vi "Enqueue Message (Single).vi"(6 "Priority Message? (F)":bool, 8 "error in (no error)":errorcluster[](array[cluster]), 9 "Message Data":variant, 10 "Message":string, 11 "Message Queue":refnum<queue>) -> (0 "error out":errorcluster[](array[cluster]), 3 "dup Message Queue":refnum<queue>)   [LabVIEW 2018, in "Message Queue.lvlib"]
doc: "For a regular message, enqueue the message. For a priority message, enqueue it at the front of the queue."
uses:
  Message Queue.lvlib
  Message Cluster.ctl
  <userlib>/NIST/NISTErrorLib/NISTErrorLib.lvlib
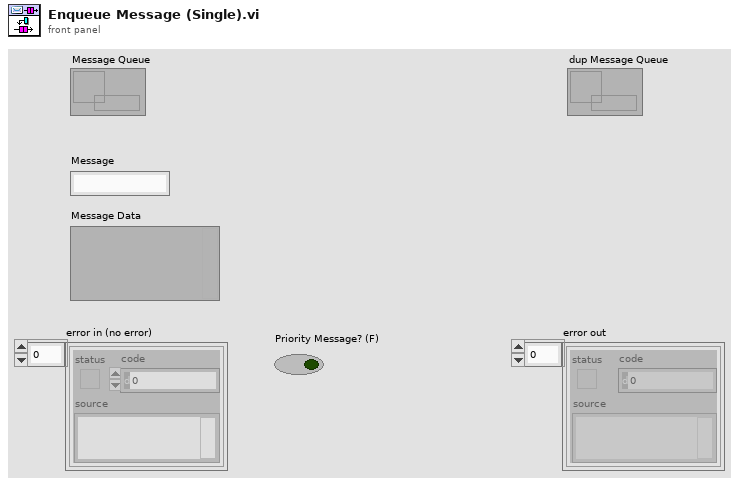
[diagram p1: front panel]
types:
  T1 = typedef "Message Queue.lvlib/Message Cluster.ctl" = cluster{"Message":string, "Message Data":variant}
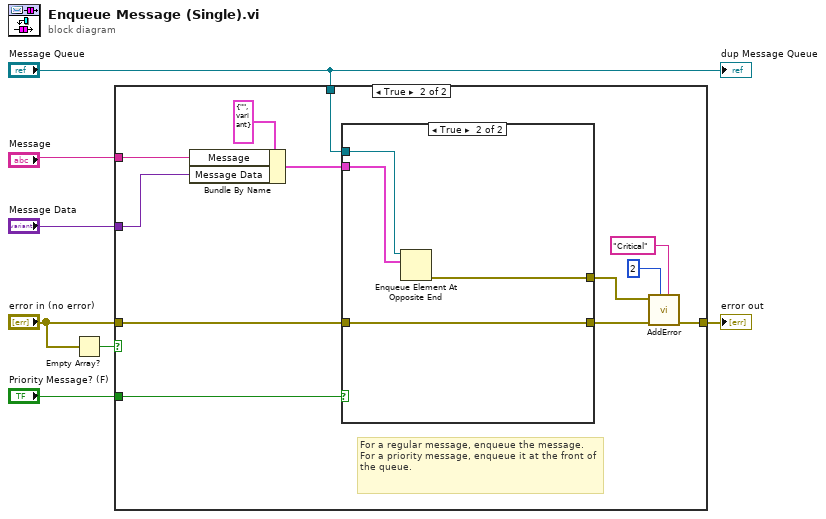
[diagram p0: block diagram]
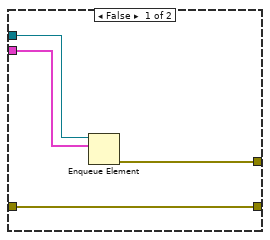
[diagram p3: hidden frame]
diagram:
  n1 = Empty Array?(array="error in (no error)") -> (empty?=w1:bool)
  n2 = case shown="True" w1 {
    tunnel: "Message" -> [_ w19]
    tunnel: "Message Data" -> [_ w18]
    tunnel: "Priority Message? (F)" -> [_ w17]
    tunnel: [w8 w12] -> w4
    tunnel: "Message Queue" -> [_ w15]
    tunnel: "error in (no error)" -> [w8 w13]
    frame False {
    }
    frame True {
      # "For a regular message, enqueue the message.  For a priority message, enqueue it at the front of the queue."
      n3 = Bundle By Name(cluster=T1 {"Message"="", "Message Data"=variant} ("Message Cluster"), "Message"=w19, "Message Data"=w18) -> (w14:T1)
      n4 = case shown="True" w17 {
        tunnel: w13 -> [w22 w25]
        tunnel: [w22 w25] -> w16
        tunnel: w15 -> [w24 w28]
        tunnel: w14 -> [w23 w27]
        tunnel: [w21 w26] -> w11
        frame False {
          n5 = Enqueue Element(queue=w24, element=w23) -> (error out=w21:errorcluster)  [unwired: 2 in, 2 out]
        }
        frame True {
          n6 = Enqueue Element At Opposite End(queue=w28, element=w27) -> (error out=w26:errorcluster)  [unwired: 2 in, 2 out]
        }
      }
      n7 = call <userlib>:"AddError.vi"("Severity"="Critical", "Priority"=u8 2, "ErrorArray In"=w16, "error in (no error)"=w11) -> ("ErrorArray Out"=w12:errorcluster[])  [unwired: 6 in, 1 out]
    }
  }
  "error out" <- w4
  "dup Message Queue" <- "Message Queue"
